vi "20 to 99.vi"(9 "Tens":string[](array[string]), 10 "Numeric":i32, 11 "0-19":string[](array[string])) -> (3 "String":string)   [LabVIEW 2013, in "Problem 17.lvlib"]
uses:
  Problem 17.lvlib
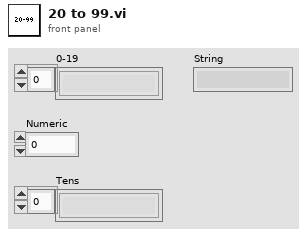
[diagram p1: front panel]
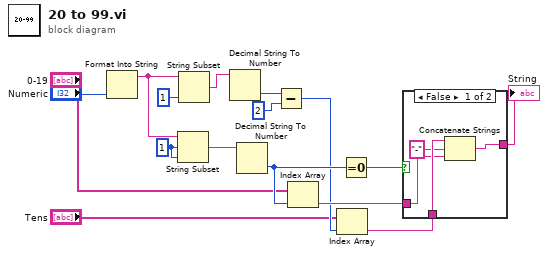
[diagram p0: block diagram]
diagram:
  w4 = 1 ("offset (0)")
  n1 = Format Into String("Numeric") -> (resulting string=w3:string)  [unwired: 3 in, 1 out]
  n2 = String Subset(string=w3, offset (0)=w4, length (rest)=w4) -> (substring=w6:string)
  n3 = String Subset(string=w3, length (rest)=1 ("length (rest)")) -> (substring=w5:string)  [unwired: 1 in]
  n4 = Decimal String To Number(string=w5) -> (number=w8:i32)  [unwired: 2 in, 1 out]
  n5 = Decimal String To Number(string=w6) -> (number=w12:i32)  [unwired: 2 in, 1 out]
  n6 = Subtract(x=w8, y=2) -> (x-y=w9:i32)
  n7 = Index Array(array="0-19", index=w12) -> (element=w15:string)
  n8 = Index Array(array="Tens", index=w9) -> (element=w14:string)
  n9 = Equal To 0?(x=w12) -> (x = 0?=w13:bool)
  n10 = case shown="False" w13 {
    tunnel: w14 -> [w20 w21]
    tunnel: w15 -> [w18 _]
    tunnel: [w19 w21] -> w16
    frame False {
      n11 = Concatenate Strings(w20, "-", w18) -> (w19:string)
    }
    frame True {
    }
  }
  "String" <- w16
